vi "Write Sample.vi"(8 "error in (no error)":errorcluster, 9 "Sample 2":refnum<class "Sample.lvclass">, 10 "Sample Line (All Closed)":T1, 11 "Sample Line in":refnum<class "Sample Line.lvclass">) -> (0 "error out":errorcluster, 3 "Sample Line out":refnum<class "Sample Line.lvclass">)   [LabVIEW 2015, in "cRIO-Carbondioxide.lvlib" / "CO2-Actor.lvlib" / "Sample Line.lvclass"]
uses:
  Sample Line.lvclass
  Controls/Sample Line State Enumerator.ctl
  subs/Sample/Sample.lvclass
  Sample Line.lvclass/Sample Line.ctl
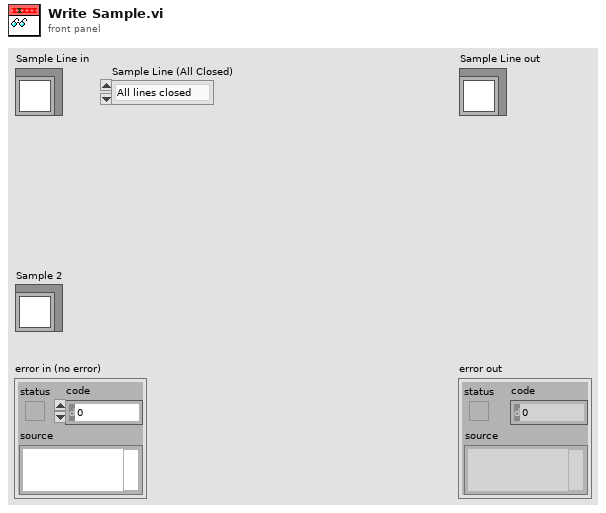
[diagram p1: front panel]
types:
  T1 = typedef "Sample Line State Enumerator.ctl" = enum16{"All lines closed", "Sample line 1.", "Sample line 2.", "Sample line 3.", "Sample line 4.", "Sample line 5.", "Out of range"}
  T2 = typedef "Sample Container.ctl" = cluster{"Sample In":refnum<k21>, "Sample Name":refnum<k21>, "Ti Cathode":refnum<k21>, "SampleQ":refnum<queue>}
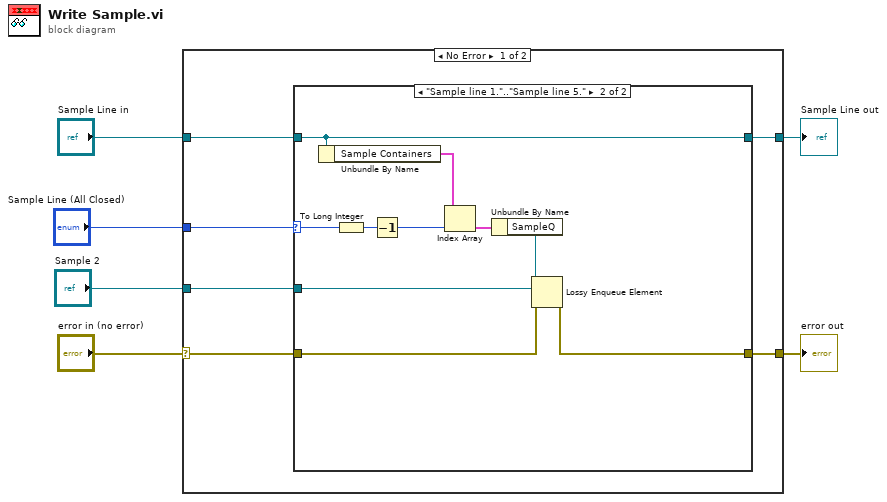
[diagram p0: block diagram]
diagram:
  n1 = case shown="No Error" "error in (no error)" {
    selector: "error in (no error)" -> [w10 w26]
    tunnel: [w9 w26] -> w5
    tunnel: [w8 w25] -> w3
    tunnel: "Sample Line in" -> [w11 w25]
    tunnel: "Sample Line (All Closed)" -> [w12 _]
    tunnel: "Sample 2" -> [w7 _]
    frame No Error {
      n2 = case shown="\"Sample line 1.\"..\"Sample line 5.\"" w12 {
        selector: w12 -> [_ w24]
        tunnel: w11 -> [w14 w21]
        tunnel: w10 -> [w13 w18]
        tunnel: [w13 w17] -> w9
        tunnel: [w14 w21] -> w8
        tunnel: w7 -> [_ w19]
        frame "All lines closed", Default {
        }
        frame "Sample line 1.".."Sample line 5." {
          n3 = Unbundle By Name(w21) -> ("Sample Containers"=w15:T2[])
          n4 = To Long Integer(number=w24) -> (32bit integer=w23:i32)
          n5 = Decrement(x=w23) -> (x-1=w16:i32)
          n6 = Index Array(array=w15, index=w16) -> (element=w22:T2)
          n7 = Unbundle By Name(w22) -> ("SampleQ"=w20:refnum<queue>)
          n8 = Lossy Enqueue Element(queue=w20, element=w19, error in (no error)=w18) -> (error out=w17:errorcluster)  [unwired: 3 out]
        }
      }
    }
    frame Error {
    }
  }
  "error out" <- w5
  "Sample Line out" <- w3
